vi "Create User Events.vi"(8 "error in (no error)":errorcluster) -> (0 "error out":errorcluster, 3 "userEvents":T1)   [LabVIEW 2019, in "HLA Custom Device Engine.lvlib" / "User Events.lvlib"]
uses:
  User Events.lvlib
  emea-ni-adg-hla-lv/src/helpers/Dictionaries/_typedefs/lv_dataType_type.ctl
  emea-ni-adg-hla-lv/src/helpers/ObjectManagement/ObjManager.lvlib
  emea-ni-adg-hla-lv/src/helpers/Dictionaries/_typedefs/parameter_type.ctl
  emea-ni-adg-hla-lv/src/helpers/Dictionaries/_typedefs/parameter_map_type.ctl
  emea-ni-adg-hla-lv/src/helpers/Dictionaries/_typedefs/attribute_type.ctl
  emea-ni-adg-hla-lv/src/helpers/Dictionaries/_typedefs/attribute_map_type.ctl
  emea-ni-adg-hla-lv/apps/generic/_typedefs/app_data.ctl
  emea-ni-adg-hla-lv/src/helpers/Dictionaries/_typedefs/interaction_type.ctl
  emea-ni-adg-hla-lv/src/helpers/Dictionaries/_typedefs/interaction_map_type.ctl
  emea-ni-adg-hla-lv/src/helpers/Dictionaries/_typedefs/object_type.ctl
  emea-ni-adg-hla-lv/src/helpers/Dictionaries/_typedefs/object_map_type.ctl
  emea-ni-adg-hla-lv/src/helpers/Dictionaries/_typedefs/instanceHandle_map_type.ctl
  objectNameNotification_type.ctl
  userEvents_type.ctl
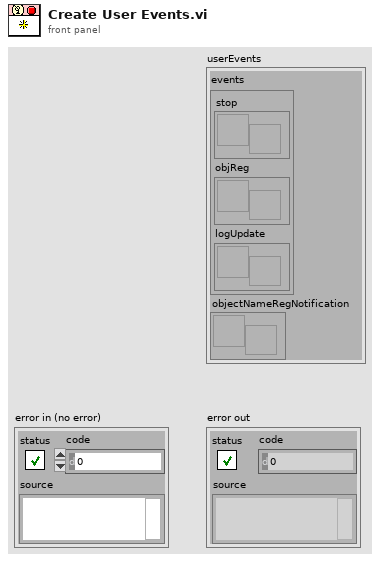
[diagram p1: front panel]
types:
  T1 = typedef "HLA Custom Device Engine.lvlib/User Events.lvlib/userEvents_type.ctl" = cluster{"events":cluster{"stop":refnum<user-event>, "objReg":refnum<user-event>, "logUpdate":refnum<user-event>}, "objectNameRegNotification":refnum<notifier>}
  T2 = typedef "HLA Custom Device Engine.lvlib/User Events.lvlib/objectNameNotification_type.ctl" = cluster{"objectInstancName":string, "success":bool}
  T3 = typedef "app_data.ctl" = cluster{"federationExecutionName":string, "federateType":string, "attrHandleSet":u64, "attrHandleValueMap":u64, "parHandleValMap":u64, "object map":T4, "interaction map":T9, "SubInstanceHandle":T13, "objectInstanceName":string, "PubInstanceHandle":T13}
  T4 = typedef "object_map_type.ctl" = map{u64, T5}
  T5 = typedef "object_type.ctl" = cluster{"handle":u64, "name":string, "attributeMap":T6, "publish":bool, "subscribe":bool}
  T6 = typedef "ObjManager.lvlib/attribute_map_type.ctl" = map{u64, T7}
  T7 = typedef "ObjManager.lvlib/attribute_type.ctl" = cluster{"handle":u64, "name":string, "dataType":T8}
  T8 = typedef "ObjManager.lvlib/lv_dataType_type.ctl" = enum16{"String", "Int32", "Double", "SpatialRVStruct", "EntityIdentifier"}
  T9 = typedef "interaction_map_type.ctl" = map{u64, T10}
  T10 = typedef "interaction_type.ctl" = cluster{"handle":u64, "name":string, "parameterMap":T11, "publish":bool, "subscribe":bool}
  T11 = typedef "ObjManager.lvlib/parameter_map_type.ctl" = map{u64, T12}
  T12 = typedef "ObjManager.lvlib/parameter_type.ctl" = cluster{"handle":u64, "name":string, "dataType":T8}
  T13 = typedef "ObjManager.lvlib/instanceHandle_map_type.ctl" = map{u64, u64}
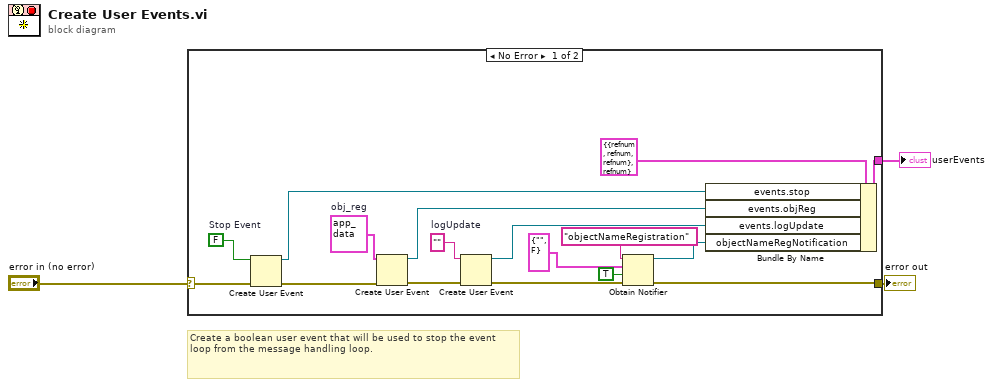
[diagram p0: block diagram]
diagram:
  # "Create a boolean user event that will be used to stop the event loop from the message handling loop."
  n1 = case shown="No Error" "error in (no error)" {
    selector: "error in (no error)" -> [w19 w21]
    tunnel: [w9 w21] -> w3
    tunnel: [w16 _] -> w1
    frame No Error {
      w12 = ""  # logUpdate
      w18 = T3 {"federationExecutionName"="", "federateType"="", "attrHandleSet"=0, "attrHandleValueMap"=0, "parHandleValMap"=0, "object map"={}, "interaction map"={}, "SubInstanceHandle"={}, "objectInstanceName"="", "PubInstanceHandle"={}}  # obj_reg
      w20 = FALSE  # Stop Event
      n2 = Create User Event(user event datatype=w20, error in=w19) -> (user event=w15:refnum<user-event>, error out=w17:errorcluster)
      n3 = Create User Event(user event datatype=w18, error in=w17) -> (user event=w14:refnum<user-event>, error out=w13:errorcluster)
      n4 = Create User Event(user event datatype=w12, error in=w13) -> (user event=w11:refnum<user-event>, error out=w10:errorcluster)
      n5 = Obtain Notifier(name (unnamed)="objectNameRegistration", notification data type=T2 {"objectInstancName"="", "success"=FALSE}, create if not found? (T)=TRUE, error in (no error)=w10) -> (notifier out=w5:refnum<notifier>, error out=w9:errorcluster)  [unwired: 1 out]
      n6 = Bundle By Name(cluster=T1 {"events"={"stop"=refnum, "objReg"=refnum, "logUpdate"=refnum}, "objectNameRegNotification"=refnum} ("userEvents"), "events.stop"=w15, "events.objReg"=w14, "events.logUpdate"=w11, "objectNameRegNotification"=w5) -> (w16:T1)
    }
    frame Error {
    }
  }
  "error out" <- w3
  "userEvents" <- w1
